vi "Gyro Yaw.vi"() -> ()   [LabVIEW 2017]
uses:
  <vilib>/Rock Robotics/WPI/ThirdParty/Sensors/navX/_TypeDefs/FRIC_navX_DeviceNumbersTypeDef.ctl
  Robot Global Data.vi
panel:
  out "Robot Yaw":dbl
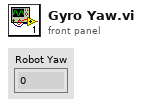
[diagram p1: front panel]
types:
  T1 = typedef "FRIC_navX_DeviceNumbersTypeDef.ctl" = enum16{"Dev0", "Dev1", "Dev2", "Dev3"}
  T2 = cluster{"Yaw":dbl, "Roll":dbl, "Pitch":dbl, "Heading":dbl, "Fused Heading":dbl}
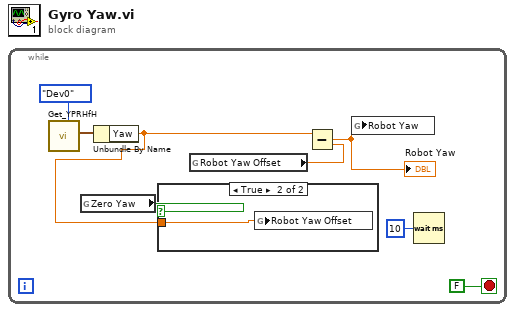
[diagram p0: block diagram]
diagram:
  n1 = while {
    stop <- FALSE stop-if-true
    n2 = call <vilib>:"Get_YPRHfH.vi"("Device Number"=FRIC_navX_DeviceNumbersTypeDef."Dev0") -> ("YRPHfH"=w7:T2)  [unwired: 10 in]
    n3 = global read "Robot Global Data.vi" "Zero Yaw"() -> (w6:bool)
    n4 = Unbundle By Name(w7) -> ("Yaw"=w4:dbl)
    n5 = case shown="True" w6 {
      tunnel: w4 -> [_ w9]
      frame False {
      }
      frame True {
        n6 = global write "Robot Global Data.vi" "Robot Yaw Offset"(w9) -> ()
      }
    }
    n7 = global read "Robot Global Data.vi" "Robot Yaw Offset"() -> (w5:dbl)
    n8 = Subtract(x=w4, y=w5) -> (x-y=w3:dbl)
    "Robot Yaw" <- w3
    n9 = global write "Robot Global Data.vi" "Robot Yaw"(w3) -> ()
    n10 = Wait (ms)(milliseconds to wait=u32 10) -> ()  [unwired: 1 out]
  }
